vi "Tools_KeyedArray Keys.vi"(7 "array in":T1) -> (2 "keys":string[](array[string]), 3 "duplicate array":T1)   [LabVIEW 2017]
doc: "Returns an array containing the keys of all the elements in <B>array in</B>."
uses:
  Tools_KeyedArray KeyedArray.ctl
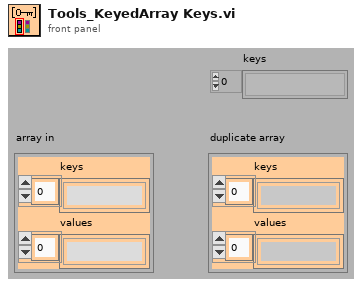
[diagram p1: front panel]
types:
  T1 = typedef "Tools_KeyedArray KeyedArray.ctl" = cluster{"keys":string[], "values":string[]}
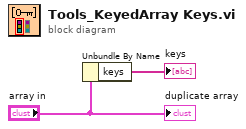
[diagram p0: block diagram]
diagram:
  n1 = Unbundle By Name("array in") -> ("keys"=→"keys":string[])
  "duplicate array" <- "array in"
